vi "fg_All Groups setup.vi"(8 "error in (no error)":errorcluster, 9 "Groups setup in":T1[](array[typedef]) {"Group region specifier cluster"."Contours"."Type" items=["No Selection", "Point", "Line", "Rectangle", "Oval", "Polygon", "Freehand Region", "Annulus", "Unused2", "Unused3", "Broken Line", "Freehand Line", "Rotated Rectangle"]}, 11 "Function":T3) -> (0 "error out":errorcluster, 1 "Groups setup out":T1[](array[typedef]) {"Group region specifier cluster"."Contours"."Type" items=["No Selection", "Point", "Line", "Rectangle", "Oval", "Polygon", "Freehand Region", "Annulus", "Unused2", "Unused3", "Broken Line", "Freehand Line", "Rotated Rectangle"]})   [LabVIEW 2017]
uses:
  Typedefs/Get-Set-Clear Control.ctl
  SubVIs/ROI Selection Interface/ROI group info cluster.ctl
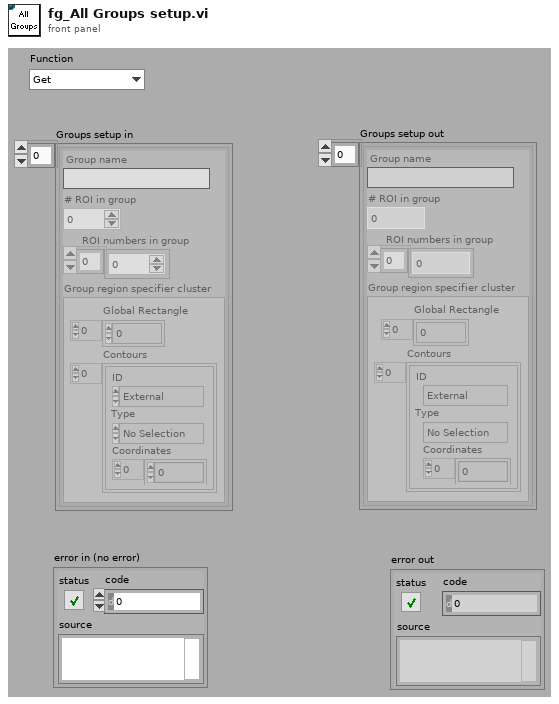
[diagram p1: front panel]
types:
  T1 = typedef "ROI group info cluster.ctl" = cluster{"Group name":string, "# ROI in group":i32, "ROI numbers in group":i32[], "Group region specifier cluster":T2}
  T2 = typedef "ROI Descriptor" = cluster{"Global Rectangle":i32[], "Contours":cluster{"ID":enum32{"External", "Internal"}, "Type":u32, "Coordinates":i32[]}[]}
  T3 = typedef "Get-Set-Clear Control.ctl" = enum16{"Get", "Set", "Clear"}
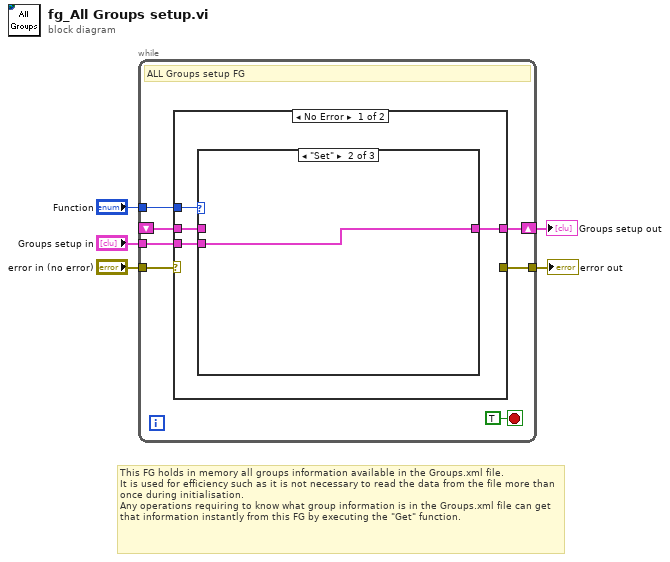
[diagram p0: block diagram]
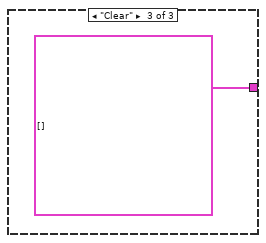
[diagram p3: hidden frame]
diagram:
  # "This FG holds in memory all groups information available in the Groups.xml file.\nIt is used for efficiency such as it is not necessary to read the data from the file more than once during initialisation.\nAny operations requiring to know what group information is in the Groups.xml file can get that information instantly from this FG by executing the \"Get\" function."
  n1 = while {
    shift-right: [w11] -> w3
    shift-left: _ -> [w9]
    tunnel: "Groups setup in" -> [w10]
    tunnel: "Function" -> [w8]
    tunnel: "error in (no error)" -> [w7]
    tunnel: [w6] -> w1
    stop <- TRUE stop-if-true
    # "ALL Groups setup FG"
    n2 = case shown="No Error" w7 {
      selector: w7 -> [_ w20]
      tunnel: [w16 _] -> w11
      tunnel: w10 -> [w15 _]
      tunnel: w9 -> [w14 _]
      tunnel: w8 -> [w13 _]
      tunnel: [_ w20] -> w6
      frame No Error {
        n3 = case shown="\"Set\"" w13 {
          tunnel: [w17 w18 T1[] [] ("Groups setup in")] -> w16
          tunnel: w15 -> [_ w18 _]
          tunnel: w14 -> [w17 _ _]
          frame "Get", Default {
          }
          frame "Set" {
          }
          frame "Clear" {
          }
        }
      }
      frame Error {
      }
    }
  }
  "Groups setup out" <- w3
  "error out" <- w1
